vi "Sys config window-Update config.vi"() -> (0 "error out":errorcluster)   [LabVIEW 2013]
uses:
  Typedefs/HW config states enum.ctl
  Visualisation/Functional Imaging Viewer/Typedefs/Get-Set-Clear Control.ctl
  Configuration code/Calibration/Globals/gl_Calibration globals.vi
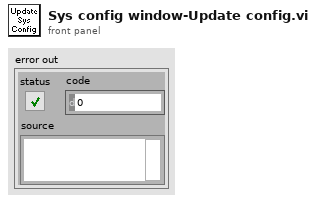
[diagram p1: front panel]
types:
  T1 = typedef "Get-Set-Clear Control.ctl" = enum16{"Get", "Set", "Clear"}
  T2 = typedef "HW config states enum.ctl" = enum16{"Load from file", "Save to file", "Write all", "Read all", "Write XY stage settings", "Write DAQ FPGA settings", "Write Control FPGA settings", "Write Phys Channels", "Clear", "Compare from file"}
  T3 = typedef "Initial config.ctl" = cluster{"System Config out":T4, "Triggers output setup":T14, "AOL Properties":T16, "Calibration settings":T17}
  T4 = typedef "Sys Configuration.ctl" = cluster{"XY Stage":T5, "DAQ FPGA":T6, "Control system":T10, "Encoder":T11, "DAQmx Chan":T12, "Computer MAC address":string, "Cam VidRec":T13, "Externalise Triggers":bool, "Laser wavelength (nm)":dbl}
  T5 = typedef "XY Stage config cluster.ctl" = cluster{"COM port":refnum<visa-resource-name>, "XY stage available":bool}
  T6 = typedef "DAQ FPGA config cluster.ctl" = cluster{"Ref":T7, "Target":T8, "Clock Freq (MHz) ":dbl, "input card type":T9, "Samples Wait after Trigger":u16, "AOD fill":u16, "StartupDelay":i32, "Slip Cycle (clock cycles)":u32, "Add Cycle":bool}
  T7 = typedef "FPGA Ref.ctl" = refnum<k20>
  T8 = typedef "nirio_resource_hc.ctl" = tag
  T9 = typedef "FPGA input type AC-DC.ctl" = enum16{"AC Card", "DC Card"}
  T10 = typedef "CTRL system config cluster.ctl" = cluster{"Ethernet opened":bool, "Ethernet Port":u32, "Ctrl FPGA available":bool, "Ctrl FPGA Clock (MHz)":dbl, "Ctrl system MAC address":string, "Control system.Network adapter name":string, "AOD 1 Amplitude":i16, "AOD 2 Amplitude":i16, "AOD 3 Amplitude":i16, "AOD 4 Amplitude":i16, "Data Time Interval (ns)":dbl, "T0 (ns)":dbl, "Ta (ns)":dbl}
  T11 = typedef "Encoder config cluster.ctl" = cluster{"IP address":string, "Port":u16, "Encoder available":bool, "Wheel radius (cm)":dbl}
  T12 = typedef "DAQmx physical channels cluster.ctl" = cluster{"Pockels AO":tag, "Hard shutter AO":tag, "PMT AOs":tag, "Power meter AI":tag}
  T13 = typedef "Cam VidRec HW config setup cluster.ctl" = cluster{"DO flag-Video record":tag, "DO flag-Trial start":tag, "VidRec available":bool}
  T14 = typedef "Triggers output setup.ctl" = T15[]
  T15 = typedef "Trigger setup element cluster.ctl" = cluster{"Name":string, "Output?":bool, "Output terminal":tag, "PXI backplane line":tag, "Pulse width (us)":u16}
  T16 = typedef "AOL Properties Cluster.ctl" = cluster{"AOD 1 thickness (mm)":dbl, "AOD 2 thickness (mm)":dbl, "AOD 3 thickness (mm)":dbl, "AOD 4 thickness (mm)":dbl, "AOD 1-2 separation (mm)":dbl, "AOD 2-3 separation (mm)":dbl, "AOD 3-4 separation (mm)":dbl, "AOL aperture (mm)":dbl, "AOL centre wavelength (nm)":dbl, "AOL centre frequency (MHz)":dbl, "skewZX":dbl, "skewZY":dbl, "magZX":dbl, "magZY":dbl, "Diffraction mode":dbl, "Crystal length (mm)":dbl, "Acoustic velocity (m/s)":dbl, "Pair deflection ratio":dbl, "AOD fill time (us)":dbl}
  T17 = typedef "Calibration settings cluster.ctl" = cluster{"Pockels cal.Zoom":u8, "Pockels cal.Dwell time (µs)":dbl}
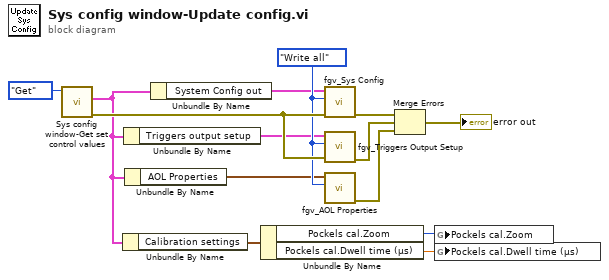
[diagram p0: block diagram]
diagram:
  w10 = HW_config_states_enum."Write all" ("Function")
  n1 = call "Sys config window-Get set control values.vi"("Function"=Get-Set-Clear_Control."Get") -> ("error out"=w13:errorcluster, "Full config"=w4:T3)  [unwired: 9 in]
  n2 = Unbundle By Name(w4) -> ("Calibration settings"=w3:T17)
  n3 = Unbundle By Name(w4) -> ("Triggers output setup"=w6:T14)
  n4 = Unbundle By Name(w4) -> ("AOL Properties"=w5:T16)
  n5 = Unbundle By Name(w4) -> ("System Config out"=w7:T4)
  n6 = Unbundle By Name(w3) -> ("Pockels cal.Zoom"=w2:u8, "Pockels cal.Dwell time (µs)"=w1:dbl)
  n7 = call "fgv_Sys Config.vi"("error in (no error)"=w13, "Function"=w10, "System Config in"=w7) -> ("error out"=w12:errorcluster)  [unwired: 7 in, 1 out]
  n8 = call "fgv_Triggers Output Setup.vi"("error in (no error)"=w13, "Function"=w10, "Triggers output setup"=w6) -> ("error out"=w11:errorcluster)  [unwired: 7 in, 1 out]
  n9 = call "fgv_AOL Properties.vi"("Function"=w10, "AOL Properties in"=w5) -> ("error out"=w9:errorcluster)  [unwired: 8 in, 1 out]
  n10 = Merge Errors(w12, w11, w9) -> (→"error out":errorcluster)
  n11 = global write "gl_Calibration globals.vi" "Pockels cal.Zoom"(w2) -> ()
  n12 = global write "gl_Calibration globals.vi" "Pockels cal.Dwell time (µs)"(w1) -> ()
